vi "AdmittanceFilter.vi"(8 "Fy":dbl, 9 "Fx":dbl, 11 "AdmittanceCoeffs":T1={"C"=1.0, "k"=1.0}) -> (0 "Delta y":dbl, 1 "Delta x":dbl)   [LabVIEW 2017, in "controllerLibrary.lvlib"]
uses:
  controllerLibrary.lvlib
  Controls/AdmittanceGains.ctl
  <vilib>/imath/engines/lvmath2/RunTimeEngine/NodeEndStatement/NIMS_NodeEndStatement_Output.vi
  <instcachedir>/0/NIMS_NodeEndStatement_Output_53EC0D466D134D7ABD903AC30B43404B.lvgen/NIMS_NodeEndStatement_Output_53EC0D466D134D7ABD903AC30B43404B_001.vi
  <vilib>/imath/engines/lvmath2/RunTimeEngine/ErrorHandling/NIMS_Finalize Error.vi
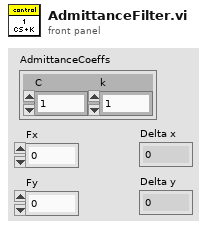
[diagram p1: front panel]
types:
  T1 = typedef "controllerLibrary.lvlib/AdmittanceGains.ctl" = cluster{"C":dbl, "k":dbl}
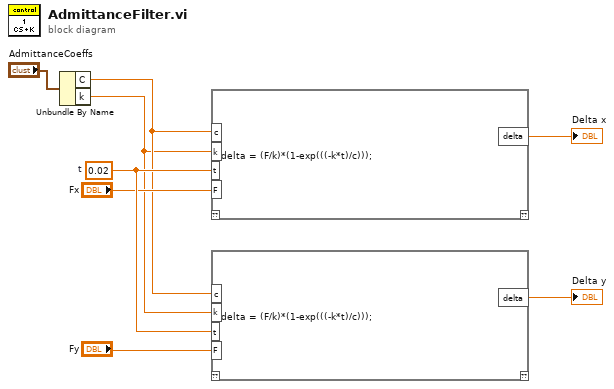
[diagram p0: block diagram]
diagram:
  w7 = 0.02  # t
  n1 = Unbundle By Name("AdmittanceCoeffs") -> ("C"=w2:dbl, "k"=w1:dbl)
  n2 = mathscript code="delta = (F/k)*(1-exp(((-k*t)/c)));"("F"="Fx", "c"=w2, "k"=w1, "t"=w7) -> ("delta"=→"Delta x":dbl)  [unwired: 1 in, 1 out]
  n3 = mathscript code="delta = (F/k)*(1-exp(((-k*t)/c)));"("F"="Fy", "c"=w2, "k"=w1, "t"=w7) -> ("delta"=→"Delta y":dbl)  [unwired: 1 in, 1 out]
